vi "PI_GCS3_Configuration_Setup_EAX.vi"(0 "System no.":i32=1 min=1 step=1, 1 "Conn. Axes":string[](array[string]), 3 "Mode of Operation":T1[](array[typedef]), 5 "error in":errorcluster, 7 "Stop refnum":refnum<vi>) -> (19 "error out":errorcluster)   [LabVIEW 2020]
doc: "Select axes which drive state is not \"Open\" and waits until enabled with EAX.\n\nWarning: Do not use this VI outside the GCS 3.0 Configuration Setup."
uses:
  Special command.llb/ModeOfOperation.ctl
panel:
  # "Enable axis for any mode of Operation.\n\nWarning: Do not use this VI outside the\nGCS 3.0 Configuration Setup."
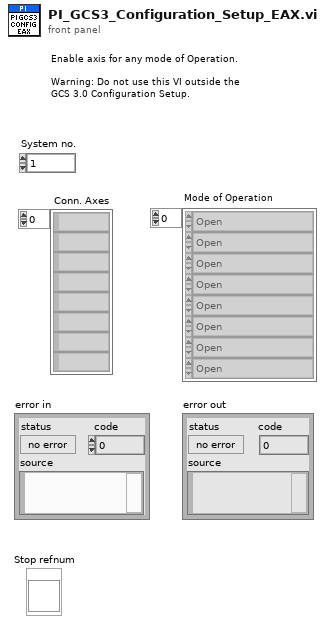
[diagram p1: front panel]
types:
  T1 = typedef "ModeOfOperation.ctl" = enum16{"Open", "Open-Loop Position", "Closed-Loop Position", "Open-Loop Velocity", "Closed-Loop Velocity", "Open-Loop Force", "Closed-Loop Force", "Step Operation"}
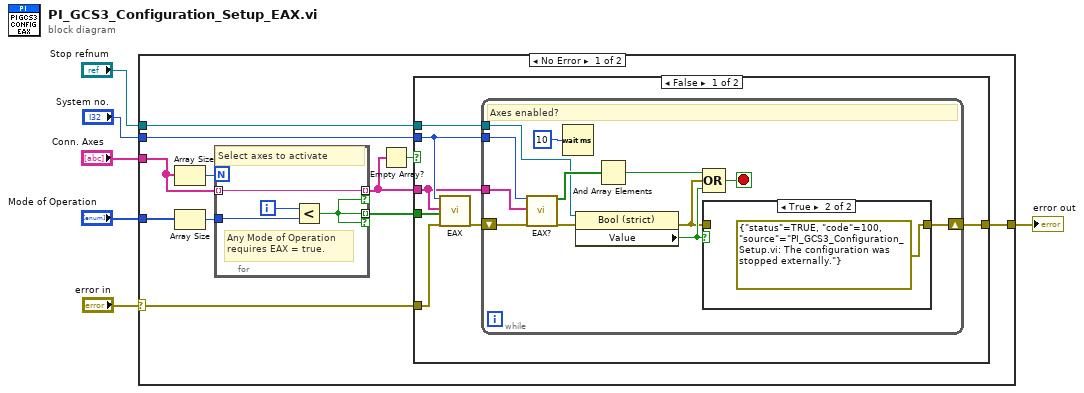
[diagram p0: block diagram]
diagram:
  n1 = case shown="No Error" "error in" {
    selector: "error in" -> [w17 w44]
    tunnel: [w16 w44] -> w5
    tunnel: "Conn. Axes" -> [w8 _]
    tunnel: "Mode of Operation" -> [w11 _]
    tunnel: "System no." -> [w15 _]
    tunnel: "Stop refnum" -> [w13 _]
    frame No Error {
      n2 = Array Size(array=w8) -> (size(s)=w12:i32)
      n3 = Array Size(array=w11) -> (size(s)=w10:i32)
      n4 = for {
        N: w12 -> [_]
        tunnel: w10 -> [w21]
        tunnel: [w18] -> w9 mode=indexing if=w18
        tunnel: w8 -> [w19] mode=indexing
        tunnel: [w19] -> w7 mode=indexing if=w18
        i -> [w20]
        # "Any Mode of Operation\nrequires EAX = true."
        # "Select axes to activate"
        n5 = Less?(x=w20, y=w21) -> (x < y?=w18:bool)
      }
      n6 = Empty Array?(array=w7) -> (empty?=w14:bool)
      n7 = case shown="False" w14 {
        tunnel: w17 -> [w28 w43]
        tunnel: [w26 w43] -> w16
        tunnel: w15 -> [w25 _]
        tunnel: w9 -> [w24 _]
        tunnel: w7 -> [w23 _]
        tunnel: w13 -> [w22 _]
        frame False {
          n8 = call "EAX.vi"("System no."=w25, "Axes to command"=w23, "Enable axis?"=w24, "error in"=w28) -> ("error out"=w27:errorcluster)  [unwired: 15 in]
          n9 = while {
            shift-right: [w34] -> w26
            shift-left: w27 -> [w40]
            tunnel: w25 -> [w38]
            tunnel: w23 -> [w37]
            tunnel: w22 -> [w35]
            stop <- w30 stop-if-true
            # "Axes enabled?"
            n10 = call "EAX?.vi"("System no."=w38, "Axes to query"=w37, "error in"=w40) -> ("Axes enabled status"=w39:bool[], "error out"=w32:errorcluster)  [unwired: 15 in]
            n11 = Wait (ms)(milliseconds to wait=u32 10) -> ()  [unwired: 1 out]
            n12 = property class="Bool (strict)"(reference=w35, error in=w32) -> (error out=w29:errorcluster, "Value"=w31:bool)  [unwired: 1 out]
            n13 = And Array Elements(Boolean array=w39) -> (logical AND=w33:bool)
            n14 = Compound Arithmetic op=OR(w33, w29, w31) -> (w30:bool)
            n15 = case shown="True" w31 {
              tunnel: [w41 errorcluster {"status"=TRUE, "code"=100, "source"="PI_GCS3_Configuration_Setup.vi: The configuration was stopped externally."} ("error out")] -> w34
              tunnel: w29 -> [w41 _]
              frame False {
              }
              frame True {
              }
            }
          }
        }
        frame True {
        }
      }
    }
    frame Error {
    }
  }
  "error out" <- w5
